vi "checkBeginFromPreparePass.vi"(6 "firstCall?":bool=TRUE, 8 "error in (no error)":errorcluster, 9 "robotKickState in":T1=enum."turn", 10 "Game in":refnum<class "Game.lvclass">, 11 "KickToSkill in":refnum<class "KickToSkill.lvclass">) -> (0 "error out":errorcluster, 1 "FromPreparePass":bool, 2 "Game out":refnum<class "Game.lvclass">, 3 "KickToSkill out":refnum<class "KickToSkill.lvclass">, 4 "state out":T1=enum."goToBackBall")   [LabVIEW 2021, in "KickToSkill.lvclass"]
uses:
  KickToSkill.lvclass
  Game_class/Game.lvclass
  Robot_class/robotKickToStates.ctl
  Game_class/Game.lvclass/Game.ctl
  Playbook_class/Playbook.lvclass/Playbook.ctl
  Team_class/Team.lvclass/Team.ctl
  5RobotsNormalGamePlay_class/5RobotsNormalGamePlay.lvclass/5RobotsNormalGamePlay.ctl
  5RobotsPassGamePlay_class/5RobotsPassGamePlay.lvclass/5RobotsPassGamePlay.ctl
  5RobotsNormalGamePlay_class/Write FromPreparePass.vi
  Playbook_class/Write offensive_plays.vi
  5RobotsNormalGamePlay_class/Read FromPreparePass.vi
  5RobotsPassGamePlay_class/Write FromPreparePass.vi
  5RobotsPassGamePlay_class/Read FromPreparePass.vi
  Game_class/Read OffensiveTeam.vi
  Team_class/Read OffensivePlay.vi
  Playbook_class/Read offensive_plays.vi
  Ally_class/Ally.lvclass
  D:/RoboIme/horie/SSL_AI/Team_class/Team.lvclass
  Playbook_class/Playbook.lvclass
  Play_class/Play.lvclass
  TestPlay_class/TestPlay.lvclass
  EnemyPossessionAtEnemyFieldPlay_class/EnemyPossessionAtEnemyFieldPlay.lvclass
  EnemyPossessionAtOurFieldPlay_class/EnemyPossessionAtOurFieldPlay.lvclass
  NormalGamePlay_class/NormalGamePlay.lvclass
  IndirectEnemyPlay_class/IndirectEnemyPlay.lvclass
  PrepareKickoffAllyPlay_class/PrepareKickoffAllyPlay.lvclass
  PrepareKickoffEnemyPlay_class/PrepareKickoffEnemyPlay.lvclass
  KickPenaltyAllyPlay_class/KickPenaltyAllyPlay.lvclass
  PreparePenaltyAllyPlay_class/PreparePenaltyAllyPlay.lvclass
  DirectEnemyPlay_class/DirectEnemyPlay.lvclass
  PreparePenaltyEnemyPlay_class/PreparePenaltyEnemyPlay.lvclass
  BallOutOfFieldPlay_class/BallOutOfFieldPlay.lvclass
  StopOffensivePlay_class/StopOffensivePlay.lvclass
  PassPlay_class/PassPlay.lvclass
  DirectKickPlay_class/DirectKickPlay.lvclass
  HaltPlay_class/HaltPlay.lvclass
  PreparePassPlay_class/PreparePassPlay.lvclass
  PassToStriker_class/PassToStriker.lvclass
  PassTo2ndStriker_class/PassTo2ndStriker.lvclass
  SimplePass_class/SimplePass.lvclass
  PrepareRollToPassPlay_class/PrepareRollToPassPlay.lvclass
  PrepareDoublePassPlay_class/PrepareDoublePassPlay.lvclass
  TableWith2ndStrikerPlay_class/TableWith2ndStrikerPlay.lvclass
  TableWithStrikerPlay_class/TableWithStrikerPlay.lvclass
  PrepareTriplePassPlay_class/PrepareTriplePassPlay.lvclass
  ABCPassPlay_class/ABCPassPlay.lvclass
  PreparePassInGame1_class/PreparePassInGame1.lvclass
  ACBPassPlay_class/ACBPassPlay.lvclass
  PrepareKeeperPassPlay_class/PrepareKeeperPassPlay.lvclass
  KeeperPassToStrikerPlay_class/KeeperPassToStrikerPlay.lvclass
  5RobotsNormalGamePlay_class/5RobotsNormalGamePlay.lvclass
  5RobotsPassGamePlay_class/5RobotsPassGamePlay.lvclass
  5RobotsKeeperGame_class/5RobotsKeeperGame.lvclass
  5PreparePassGamePlay_class/5PreparePassGamePlay.lvclass
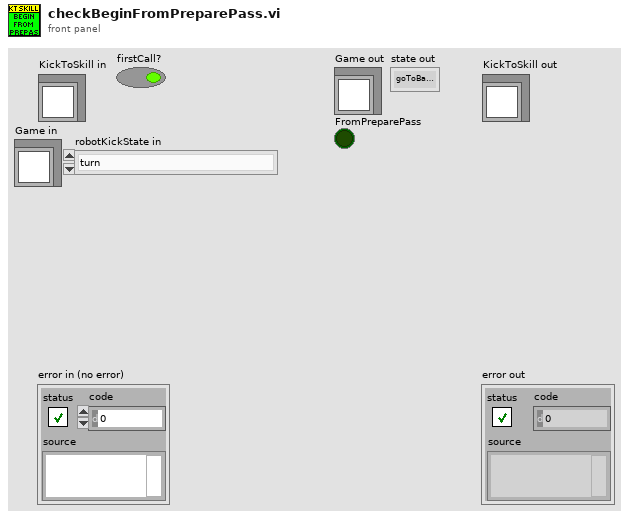
[diagram p1: front panel]
types:
  T1 = typedef "robotKickToStates.ctl" = enum16{"shootFromDirect", "avoidCollideBall", "goToBackBall", "none", "walk", "turn", "oldKickToShoot", "oldKickToGoToBackBall", "shoot"}
  T2 = typedef "offensive_plays.ctl" = cluster{"Play":refnum<class "Play.lvclass">, "TestPlay":refnum<class "TestPlay.lvclass">, "EnemyPossessionAtEnemyFieldPlay":refnum<class "EnemyPossessionAtEnemyFieldPlay.lvclass">, "EnemyPossessionAtOurFieldPlay":refnum<class "EnemyPossessionAtOurFieldPlay.lvclass">, "NormalGamePlay":refnum<class "NormalGamePlay.lvclass">, "IndirectEnemyPlay":refnum<class "IndirectEnemyPlay.lvclass">, "PrepareKickoffAllyPlay":refnum<class "PrepareKickoffAllyPlay.lvclass">, "PrepareKickoffEnemyPlay":refnum<class "PrepareKickoffEnemyPlay.lvclass">, "KickPenaltyAllyPlay":refnum<class "KickPenaltyAllyPlay.lvclass">, "PreparePenaltyAllyPlay":refnum<class "PreparePenaltyAllyPlay.lvclass">, "DirectEnemyPlay":refnum<class "DirectEnemyPlay.lvclass">, "PreparePenaltyEnemyPlay":refnum<class "PreparePenaltyEnemyPlay.lvclass">, "BallOutOfFieldPlay":refnum<class "BallOutOfFieldPlay.lvclass">, "StopOffensivePlay":refnum<class "StopOffensivePlay.lvclass">, "PassPlay":refnum<class "PassPlay.lvclass">, "DirectKickPlay":refnum<class "DirectKickPlay.lvclass">, "HaltPlay":refnum<class "HaltPlay.lvclass">, "PreparePassPlay":refnum<class "PreparePassPlay.lvclass">, "PassToStrikerPlay":refnum<class "PassToStriker.lvclass">, "PassTo2ndStrikerPlay":refnum<class "PassTo2ndStriker.lvclass">, "SimplePassPlay":refnum<class "SimplePass.lvclass">, "PrepareRollToPassPlay":refnum<class "PrepareRollToPassPlay.lvclass">, "PrepareDoublePassPlay":refnum<class "PrepareDoublePassPlay.lvclass">, "TableWith2ndStrikerPlay":refnum<class "TableWith2ndStrikerPlay.lvclass">, "TableWithStrikerPlay":refnum<class "TableWithStrikerPlay.lvclass">, "PrepareTriplePassPlay":refnum<class "PrepareTriplePassPlay.lvclass">, "ABCPassPlay":refnum<class "ABCPassPlay.lvclass">, "PreparePassInGame1":refnum<class "PreparePassInGame1.lvclass">, "ACBPassPlay":refnum<class "ACBPassPlay.lvclass">, "PrepareKeeperPassPlay":refnum<class "PrepareKeeperPassPlay.lvclass">, "KeeperPassToStrikerPlay":refnum<class "KeeperPassToStrikerPlay.lvclass">, "SimplePass":refnum<class "SimplePass.lvclass">, "SimplePass 2":refnum<class "SimplePass.lvclass">, "5RobotsNormalGamePlay":refnum<class "5RobotsNormalGamePlay.lvclass">, "5RobotsPassGamePlay":refnum<class "5RobotsPassGamePlay.lvclass">, "5RobotsKeeperGame":refnum<class "5RobotsKeeperGame.lvclass">, "5PreparePassGamePlay":refnum<class "5PreparePassGamePlay.lvclass">}
  T3 = typedef "OffensivePlay.ctl" = enum16{"5RobotsPassGamePlay", "5PreparePassGame", "5RobotsKeeperGame", "KeeperPassToStriker", "5RobotsNormalGamePlay", "PrepareKeeperPass", "ACBPass", "ABCPass", "PrepareTriplePass", "TableWithStriker", "TableWith2ndStrikerPlay", "PrepareDoublePass", "PrepareRollToPass", "SimplePass", "PreparePass", "PassToStriker", "BallOutOfField", "PassTo2ndStriker", "StopOffensive", "Prepare Penalty Enemy", "EnemyPossessionAtEnemyField", "EnemyPossesionAtOurField", "TestPlay", "PreparePenaltyAlly", "KickPenaltyAlly", "PrepareKickoffAlly", "PrepareKickoffEnemy", "IndirectEnemy", "DirectEnemy", "PreparePassInGame1", "NormalGame", "DirectKick", "Pass", "Halt", "Timeout", "PassPlay", "PenaltyEnemy"}
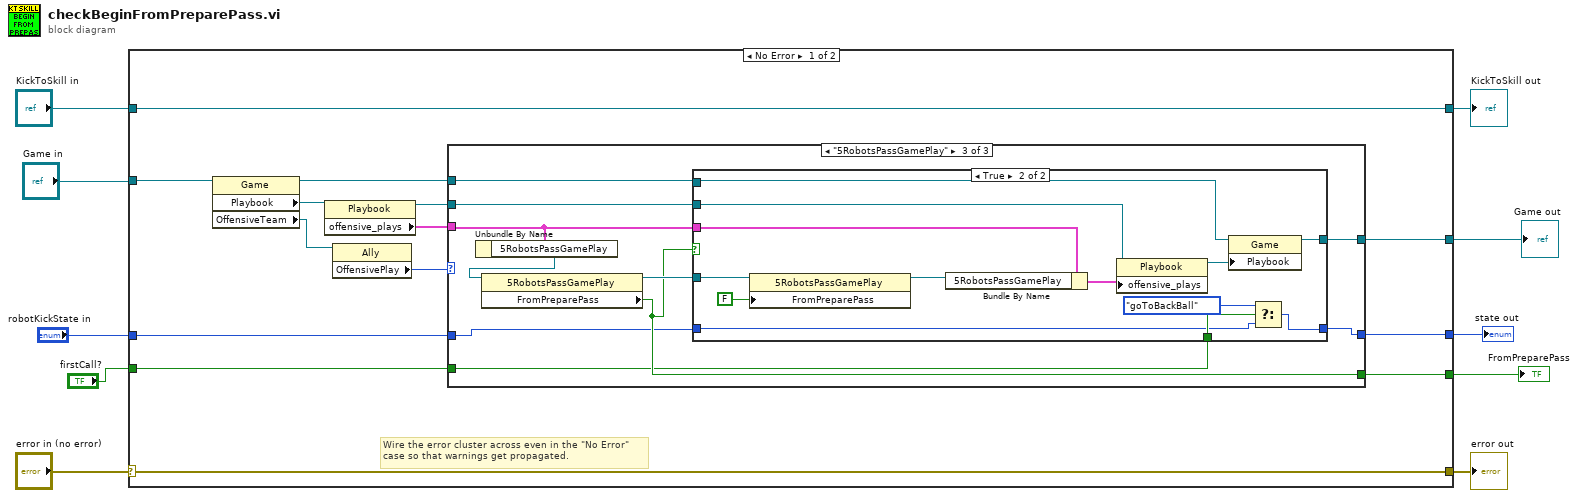
[diagram p0: block diagram]
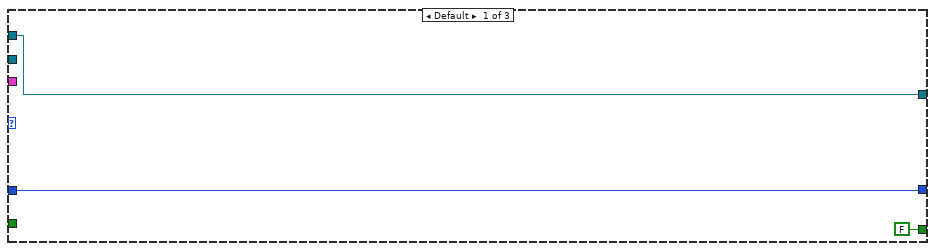
[diagram p2: hidden frame]
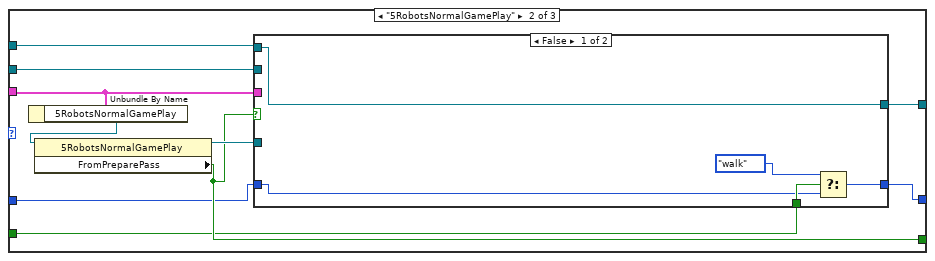
[diagram p3: hidden frame]
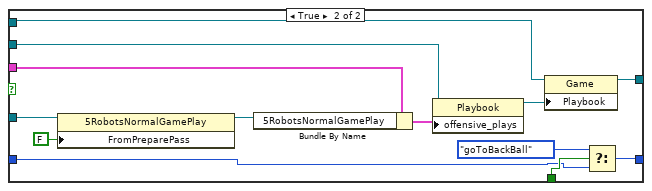
[diagram p4: hidden frame]
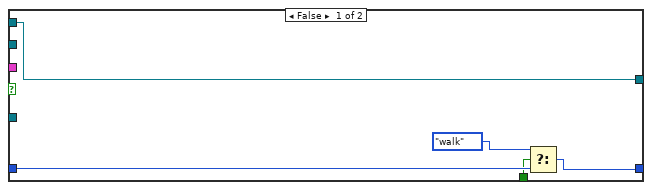
[diagram p5: hidden frame]
diagram:
  n1 = case shown="No Error" "error in (no error)" {
    selector: "error in (no error)" -> [w23 w85]
    tunnel: [w23 w85] -> w9
    tunnel: [w24 w84] -> w7
    tunnel: "KickToSkill in" -> [w24 w84]
    tunnel: "Game in" -> [w22 _]
    tunnel: [w21 _] -> w5
    tunnel: [w20 _] -> w4
    tunnel: "robotKickState in" -> [w19 _]
    tunnel: [w18 _] -> w3
    tunnel: "firstCall?" -> [w17 _]
    frame No Error {
      # "Wire the error cluster across even in the \"No Error\"\ncase so that warnings get propagated."
      n2 = property class="Game"(reference=w22) -> (reference out=w11:refnum<class "Game.lvclass">, "Playbook"=w16:refnum<class "Playbook.lvclass">, "OffensiveTeam"=w14:refnum<class "Ally.lvclass">)  [unwired: 1 in, 1 out]
      n3 = property class="Playbook"(reference=w16) -> (reference out=w12:refnum<class "Playbook.lvclass">, "offensive_plays"=w15:T2)  [unwired: 1 in, 1 out]
      n4 = property class="Ally"(reference=w14) -> ("OffensivePlay"=w13:T3)  [unwired: 1 in, 2 out]
      n5 = case shown="\"5RobotsPassGamePlay\"" w13 {
        tunnel: w15 -> [_ w35 w63]
        tunnel: [FALSE ("FromPreparePass") w31 w59] -> w21
        tunnel: w12 -> [_ w34 w62]
        tunnel: w11 -> [w27 w33 w61]
        tunnel: [w27 w32 w60] -> w20
        tunnel: [w25 w30 w58] -> w18
        tunnel: w19 -> [w25 w29 w57]
        tunnel: w17 -> [_ w28 w56]
        frame Default {
        }
        frame "5RobotsNormalGamePlay" {
          n6 = Unbundle By Name(w35) -> ("5RobotsNormalGamePlay"=w36:refnum<class "5RobotsNormalGamePlay.lvclass">)
          n7 = property class="5RobotsNormalGamePlay"(reference=w36) -> (reference out=w37:refnum<class "5RobotsNormalGamePlay.lvclass">, "FromPreparePass"=w31:bool)  [unwired: 1 in, 1 out]
          n8 = case shown="False" w31 {
            tunnel: w37 -> [_ w55]
            tunnel: w35 -> [_ w53]
            tunnel: w34 -> [_ w51]
            tunnel: w33 -> [w42 w49]
            tunnel: [w42 w47] -> w32
            tunnel: [w39 w45] -> w30
            tunnel: w29 -> [w40 w43]
            tunnel: w28 -> [w41 w44]
            frame False {
              n9 = Select(t=robotKickToStates."walk" ("robotKickState"), s=w41, f=w40) -> (s? t:f=w39:T1)
            }
            frame True {
              n10 = property class="5RobotsNormalGamePlay"(reference=w55, "FromPreparePass"=FALSE) -> (reference out=w52:refnum<class "5RobotsNormalGamePlay.lvclass">)  [unwired: 1 in, 1 out]
              n11 = Bundle By Name(cluster=w53, "5RobotsNormalGamePlay"=w52) -> (w50:T2)
              n12 = property class="Playbook"(reference=w51, "offensive_plays"=w50) -> (reference out=w48:refnum<class "Playbook.lvclass">)  [unwired: 1 in, 1 out]
              n13 = property class="Game"(reference=w49, "Playbook"=w48) -> (reference out=w47:refnum<class "Game.lvclass">)  [unwired: 1 in, 1 out]
              n14 = Select(t=robotKickToStates."goToBackBall" ("state in"), s=w44, f=w43) -> (s? t:f=w45:T1)
            }
          }
        }
        frame "5RobotsPassGamePlay" {
          n15 = Unbundle By Name(w63) -> ("5RobotsPassGamePlay"=w64:refnum<class "5RobotsPassGamePlay.lvclass">)
          n16 = property class="5RobotsPassGamePlay"(reference=w64) -> (reference out=w65:refnum<class "5RobotsPassGamePlay.lvclass">, "FromPreparePass"=w59:bool)  [unwired: 1 in, 1 out]
          n17 = case shown="True" w59 {
            tunnel: w65 -> [_ w83]
            tunnel: w63 -> [_ w81]
            tunnel: w62 -> [_ w79]
            tunnel: w61 -> [w70 w77]
            tunnel: [w70 w75] -> w60
            tunnel: [w67 w72] -> w58
            tunnel: w57 -> [w69 w71]
            tunnel: w56 -> [w68 w74]
            frame False {
              n18 = Select(t=robotKickToStates."walk" ("robotKickState"), s=w68, f=w69) -> (s? t:f=w67:T1)
            }
            frame True {
              n19 = property class="5RobotsPassGamePlay"(reference=w83, "FromPreparePass"=FALSE) -> (reference out=w80:refnum<class "5RobotsPassGamePlay.lvclass">)  [unwired: 1 in, 1 out]
              n20 = Bundle By Name(cluster=w81, "5RobotsPassGamePlay"=w80) -> (w78:T2)
              n21 = property class="Playbook"(reference=w79, "offensive_plays"=w78) -> (reference out=w76:refnum<class "Playbook.lvclass">)  [unwired: 1 in, 1 out]
              n22 = property class="Game"(reference=w77, "Playbook"=w76) -> (reference out=w75:refnum<class "Game.lvclass">)  [unwired: 1 in, 1 out]
              n23 = Select(t=robotKickToStates."goToBackBall" ("state in"), s=w74, f=w71) -> (s? t:f=w72:T1)
            }
          }
        }
      }
    }
    frame Error {
    }
  }
  "error out" <- w9
  "KickToSkill out" <- w7
  "Game out" <- w4
  "FromPreparePass" <- w5
  "state out" <- w3
